vi "CalculateDeltas_GetEveryNthRow.vi"(0 "Input 2D Numeric Array":dbl[][](array[numeric]), 3 "First Row's Index":i32, 5 "Get every n-th Row:":i32) -> (6 "Output Rows":dbl[][](array[numeric]))   [LabVIEW 2013]
doc: "This SubVI takes a 2D numeric array as input and extracts every Nth row from it, beginning with the Row with Index = \"First Row's Index\" (zero-indexed)."
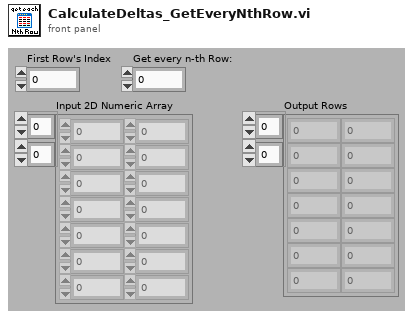
[diagram p1: front panel]
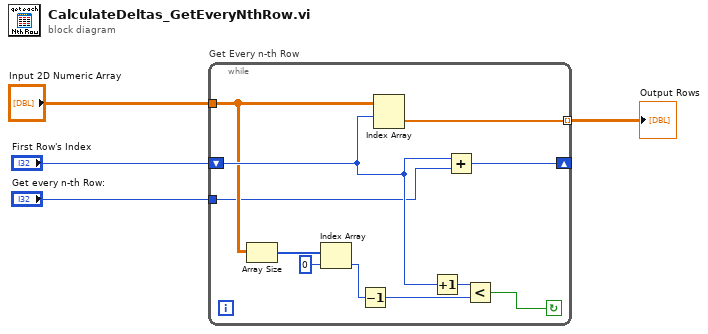
[diagram p0: block diagram]
diagram:
  n1 = while "Get Every n-th Row" {
    tunnel: "Input 2D Numeric Array" -> [w6]
    shift-right: [w13] -> _
    shift-left: "First Row's Index" -> [w11]
    tunnel: [w12] -> w4 mode=indexing
    tunnel: "Get every n-th Row:" -> [w5]
    stop <- w14 continue-if-true
    n2 = Array Size(array=w6) -> (size(s)=w7:i32[])
    n3 = Index Array "Index Array"(array=w7, index=0) -> (element=w9:i32)
    n4 = Decrement(x=w9) -> (x-1=w8:i32)
    n5 = Index Array "Index Array"(array=w6, index (row)=w11) -> (element=w12:dbl[])  [unwired: 1 in]
    n6 = Increment(x=w11) -> (x+1=w10:i32)
    n7 = Add(x=w11, y=w5) -> (x+y=w13:i32)
    n8 = Less?(x=w10, y=w8) -> (x < y?=w14:bool)
  }
  "Output Rows" <- w4
